vi "Update Menus.vi"(8 "error in (no error)":errorcluster, 10 "Left Menu":refnum<vi>, 11 "Right Menu":refnum<vi>) -> (0 "error out":errorcluster)   [LabVIEW 2020]
doc: "This VI updates the ATM Menus."
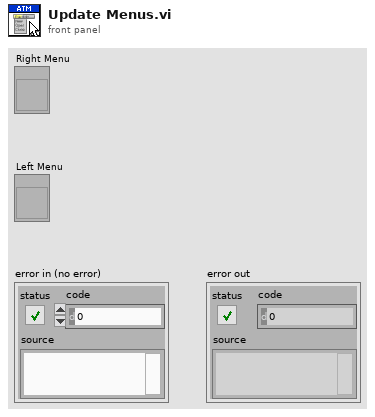
[diagram p1: front panel]
types:
  T1 = cluster{"RFS String":string, "RFS String 2":string, "RFS String 3":string}
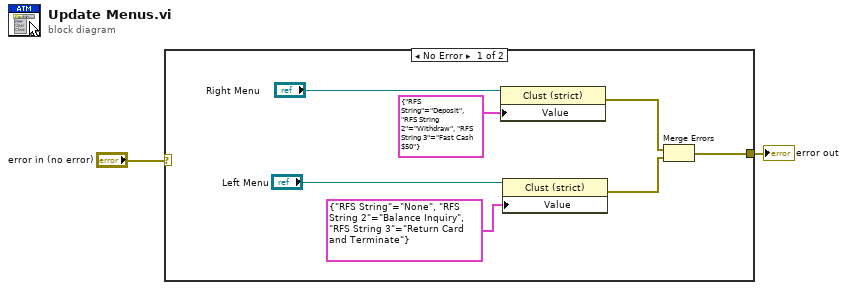
[diagram p0: block diagram]
diagram:
  n1 = case shown="No Error" "error in (no error)" {
    selector: "error in (no error)" -> [_ w10]
    tunnel: [w3 w10] -> w2
    frame No Error {
      n2 = property class="Clust (strict)"(reference="Right Menu", "Value"=T1 {"RFS String"="Deposit", "RFS String 2"="Withdraw", "RFS String 3"="Fast Cash $50"}) -> (error out=w5:errorcluster)  [unwired: 1 in, 1 out]
      n3 = property class="Clust (strict)"(reference="Left Menu", "Value"=T1 {"RFS String"="None", "RFS String 2"="Balance Inquiry", "RFS String 3"="Return Card and Terminate"}) -> (error out=w4:errorcluster)  [unwired: 1 in, 1 out]
      n4 = Merge Errors(w5, w4) -> (w3:errorcluster)
    }
    frame Error {
    }
  }
  "error out" <- w2
